vi "Get Hardware Data.vi"(8 "error in (no error)":errorcluster, 11 "Device Ref in":T1 format="%.0x") -> (0 "error out":errorcluster, 2 "Hardware":T2={"Switch Device"="", "DMM Device"="PXI1Slot6", "DMM -> Switch Trigger"=0, "Switch -> DMM Trigger"=0, "Sample Interval (sec)"=0.1, "Current Samples"=1, "Current Limit"=1.2, "Current Resolution"=5.5, "Auto-Read"=FALSE, "Keep Values"=FALSE} {"Current Resolution" items=["3 1/2"=3.5, "4 1/2"=4.5, "5 1/2"=5.5, "6 1/2"=6.5, "7 1/2"=7.5]; "Sample Interval (sec)" format="%.2f"}, 3 "Item Ref out":T1 format="%.0x")   [LabVIEW 2011, in "Switch-DMM Custom Device.lvlib"]
uses:
  Switch-DMM Custom Device.lvlib
  Controls/Hardware.ctl
  <instrlib>/niDMM/nidmm.llb/niDMM Resolution in Digits.ctl
  <vilib>/NI Veristand/Custom Device API/Custom Device Item Ref.ctl
  Controls/Globals.vi
  <vilib>/NI Veristand/Custom Device API/Get Item Property (String).vi
  <vilib>/NI Veristand/Custom Device API/Get Item Property (U16).vi
  <vilib>/NI Veristand/Custom Device API/Get Item Property (Double).vi
  <vilib>/NI Veristand/Custom Device API/Get Item Property (I32).vi
  <vilib>/NI Veristand/Custom Device API/Get Item Property (Boolean).vi
  <vilib>/NI Veristand/Custom Device API/Custom Device API.lvlib
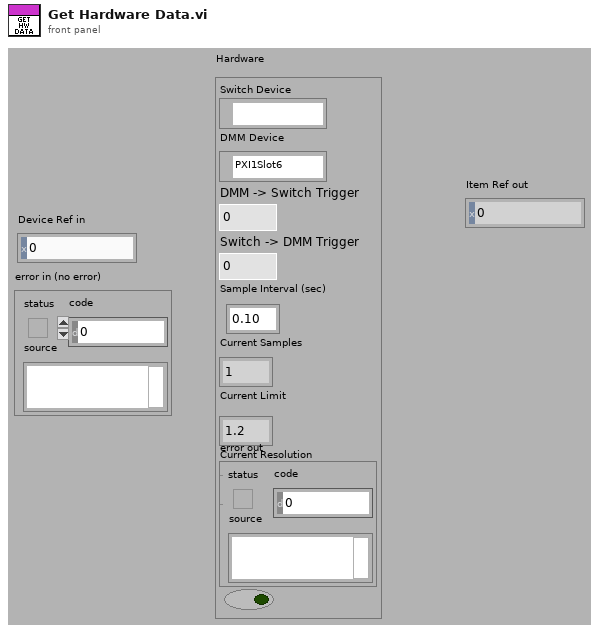
[diagram p1: front panel]
types:
  T1 = typedef "Custom Device API.lvlib/Custom Device Item Ref.ctl" = u64
  T2 = typedef "Switch-DMM Custom Device.lvlib/Hardware.ctl" = cluster{"Switch Device":refnum<k15>, "DMM Device":refnum<k15>, "DMM -> Switch Trigger":u16, "Switch -> DMM Trigger":u16, "Sample Interval (sec)":dbl, "Current Samples":i32, "Current Limit":dbl, "Current Resolution":T3, "Auto-Read":bool, "Keep Values":bool}
  T3 = typedef "niDMM Resolution in Digits.ctl" = dbl
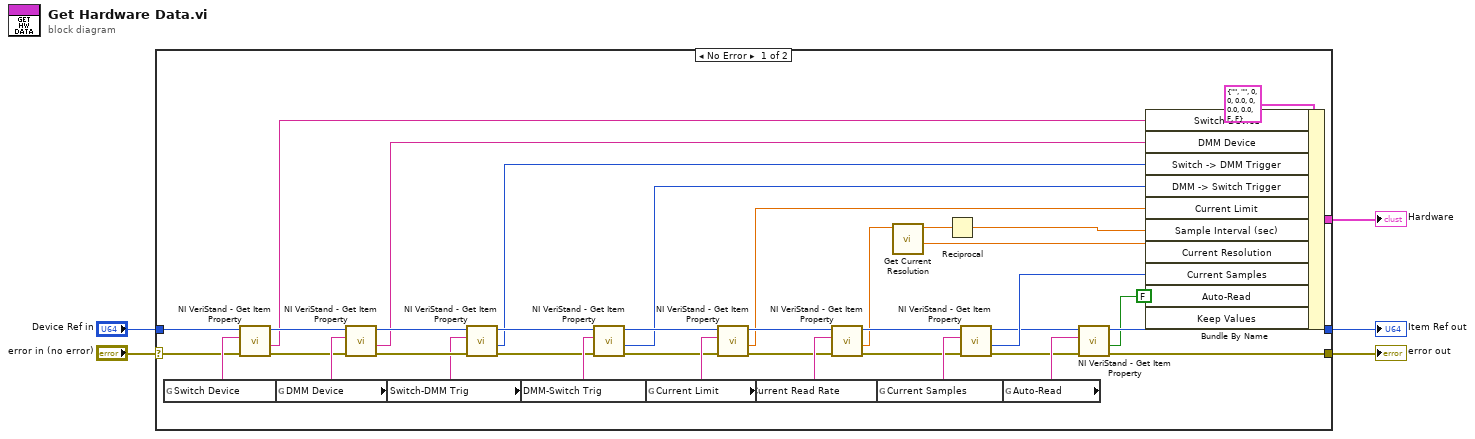
[diagram p0: block diagram]
diagram:
  n1 = case shown="No Error" "error in (no error)" {
    selector: "error in (no error)" -> [w20 w46]
    tunnel: [w45 _] -> w5
    tunnel: "Device Ref in" -> [w27 w47]
    tunnel: [w18 w47] -> w3
    tunnel: [w17 w46] -> w2
    frame No Error {
      n2 = global read "Globals.vi" "Switch Device"() -> (w28:string)
      n3 = call-poly <vilib>:"NI VeriStand - Get Item Property.vi"("error in (no error)"=w20, "Property Name"=w28, "Item Ref in"=w27) -> ("error out"=w30:errorcluster, "Value"=w26:string, "Item Ref out"=w29:T1)  [unwired: 5 in, 1 out]
      n4 = global read "Globals.vi" "DMM Device"() -> (w31:string)
      n5 = call-poly <vilib>:"NI VeriStand - Get Item Property.vi"("error in (no error)"=w30, "Property Name"=w31, "Item Ref in"=w29) -> ("error out"=w33:errorcluster, "Value"=w25:string, "Item Ref out"=w34:T1)  [unwired: 5 in, 1 out]
      n6 = global read "Globals.vi" "Switch-DMM Trig"() -> (w32:string)
      n7 = call-poly <vilib>:"NI VeriStand - Get Item Property.vi"("error in (no error)"=w33, "Property Name"=w32, "Item Ref in"=w34) -> ("error out"=w36:errorcluster, "Value"=w24:u16, "Item Ref out"=w35:T1)  [unwired: 5 in, 1 out]
      n8 = global read "Globals.vi" "DMM-Switch Trig"() -> (w37:string)
      n9 = call-poly <vilib>:"NI VeriStand - Get Item Property.vi"("error in (no error)"=w36, "Property Name"=w37, "Item Ref in"=w35) -> ("error out"=w39:errorcluster, "Value"=w23:u16, "Item Ref out"=w38:T1)  [unwired: 5 in, 1 out]
      n10 = global read "Globals.vi" "Current Limit"() -> (w42:string)
      n11 = call-poly <vilib>:"NI VeriStand - Get Item Property.vi"("error in (no error)"=w39, "Property Name"=w42, "Item Ref in"=w38) -> ("error out"=w41:errorcluster, "Value"=w22:dbl, "Item Ref out"=w40:T1)  [unwired: 5 in, 1 out]
      n12 = global read "Globals.vi" "Current Read Rate"() -> (w43:string)
      n13 = call-poly <vilib>:"NI VeriStand - Get Item Property.vi"("error in (no error)"=w41, "Property Name"=w43, "Item Ref in"=w40) -> ("error out"=w13:errorcluster, "Value"=w8:dbl, "Item Ref out"=w12:T1)  [unwired: 5 in, 1 out]
      n14 = global read "Globals.vi" "Current Samples"() -> (w14:string)
      n15 = call "Get Current Resolution.vi"("Current Rate in"=w8) -> ("Resolution in Digits"=w6:T3, "Current Rate out"=w7:dbl)  [unwired: 9 in]
      n16 = Reciprocal(x=w7) -> (1/x=w21:dbl)
      n17 = call-poly <vilib>:"NI VeriStand - Get Item Property.vi"("error in (no error)"=w13, "Property Name"=w14, "Item Ref in"=w12) -> ("error out"=w9:errorcluster, "Value"=w11:i32, "Item Ref out"=w10:T1)  [unwired: 5 in, 1 out]
      n18 = global read "Globals.vi" "Auto-Read"() -> (w19:string)
      n19 = call-poly <vilib>:"NI VeriStand - Get Item Property.vi"("error in (no error)"=w9, "Property Name"=w19, "Item Ref in"=w10) -> ("error out"=w17:errorcluster, "Value"=w16:bool, "Item Ref out"=w18:T1)  [unwired: 5 in, 1 out]
      n20 = Bundle By Name(cluster=T2 {"Switch Device"="", "DMM Device"="", "DMM -> Switch Trigger"=0, "Switch -> DMM Trigger"=0, "Sample Interval (sec)"=0.0, "Current Samples"=0, "Current Limit"=0.0, "Current Resolution"=0.0, "Auto-Read"=FALSE, "Keep Values"=FALSE} ("Hardware"), "Switch Device"=w26, "DMM Device"=w25, "Switch -> DMM Trigger"=w24, "DMM -> Switch Trigger"=w23, "Current Limit"=w22, "Sample Interval (sec)"=w21, "Current Resolution"=w6, "Current Samples"=w11, "Auto-Read"=w16, "Keep Values"=FALSE) -> (w45:T2)
    }
    frame Error {
    }
  }
  "Hardware" <- w5
  "Item Ref out" <- w3
  "error out" <- w2
